vi "Max Lines.vi"(10 "max lines":i32, 11 "String in":string) -> (3 "string out":string)   [LabVIEW 2015, in "Utilities 1.lvlib"]
uses:
  Utilities 1.lvlib
panel:
  out "array":string[](array[string])
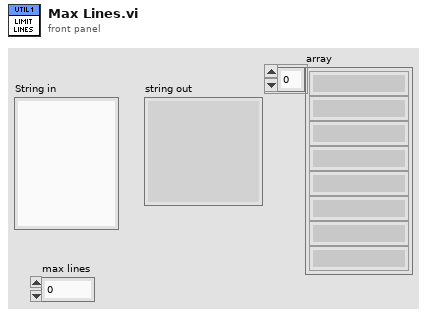
[diagram p1: front panel]
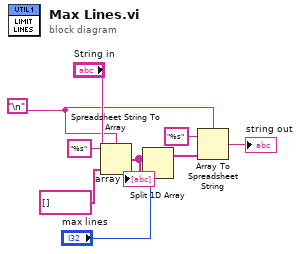
[diagram p0: block diagram]
diagram:
  w1 = "\n"
  n1 = Spreadsheet String To Array(delimiter (Tab)=w1, format string="%s", spreadsheet string="String in", array type (2D Dbl)=string[] []) -> (array=w5:string[])
  "array" <- w5
  n2 = Split 1D Array(array=w5, index="max lines") -> (first subarray=w7:string[])  [unwired: 1 out]
  n3 = Array To Spreadsheet String(delimiter (Tab)=w1, array=w7, 3:"%s" ("format string")) -> (spreadsheet string=→"string out":string)
